vi "Crop (Rectangle Points ARGB).vi"(6 "Point B":T3, 8 "error in (no error)":errorcluster, 9 "Point A":T2, 10 "ARGB Image Destination in":T4, 11 "ARGB Image Source in":T4) -> (0 "error out":errorcluster, 1 "Computed Size":T1, 3 "ARGB Image Destination":T4)   [LabVIEW 2020, in "image.lvlib"]
doc: "Crop the Source Image region specified by two corner points into the Destination Image."
uses:
  image.lvlib
  ARGB Image.ctl
  common/Image Point (Float).ctl
  common/Image Point (Integer).ctl
  common/Image Size (Integer).ctl
  2dc01dea-48f6-4df4-8727-934e95e7e307.vi
  <vilib>/Utility/error.llb/Error Cluster From Error Code.vi
  common/common.lvlib
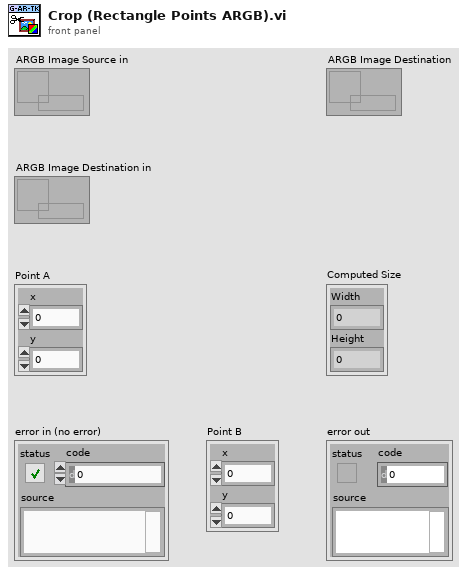
[diagram p1: front panel]
types:
  T1 = typedef "common.lvlib/Image Size (Integer).ctl" = cluster{"Width":u16, "Height":u16}
  T2 = typedef "common.lvlib/Image Point (Integer).ctl" = cluster{"x":i32, "y":i32}
  T3 = typedef "common.lvlib/Image Point (Float).ctl" = cluster{"x":dbl, "y":dbl}
  T4 = typedef "image.lvlib/ARGB Image.ctl" = refnum<data-value>
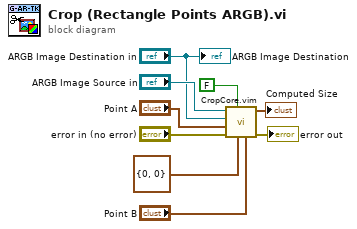
[diagram p0: block diagram]
diagram:
  n1 = call "CropCore.vim"("Other Point"="Point B", "Size"=T1 {"Width"=0, "Height"=0}, "Use Size"=FALSE, "error in (no error)"="error in (no error)", "Origin"="Point A", "Dst"="ARGB Image Destination in", "Src"="ARGB Image Source in") -> ("error out"=→"error out":errorcluster, "Computed Size"=→"Computed Size":T1)  [unwired: 3 in]
  "ARGB Image Destination" <- "ARGB Image Destination in"
